vi "SW_Fire_TTL_at_start_universal.vi"(6 "TTL port(s) config to fire":u8, 7 "TTL pulse length, ms":dbl=250.0 format="%#_13g", 8 "error in (no error)":errorcluster, 9 "Serial Port In":refnum<visa-resource-name>="COM3", 10 "Close VISA (T)":bool=TRUE, 11 "Start/stop signaling (F)":bool) -> (0 "error out":errorcluster, 1 "Serial Port Out":refnum<visa-resource-name>="COM3", 3 "Time spent to process command, ms":dbl=250.0)   [LabVIEW 2016]
doc: "Fires TTL High to the TTL2 output for ~250 ms (default)."
uses:
  <vilib>/Instr/_visa.llb/VISA Flush IO Buffer Mask.ctl
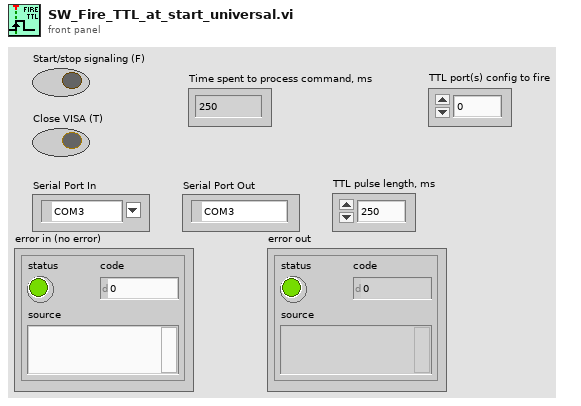
[diagram p1: front panel]
types:
  T1 = typedef "VISA Flush IO Buffer Mask.ctl" = u16
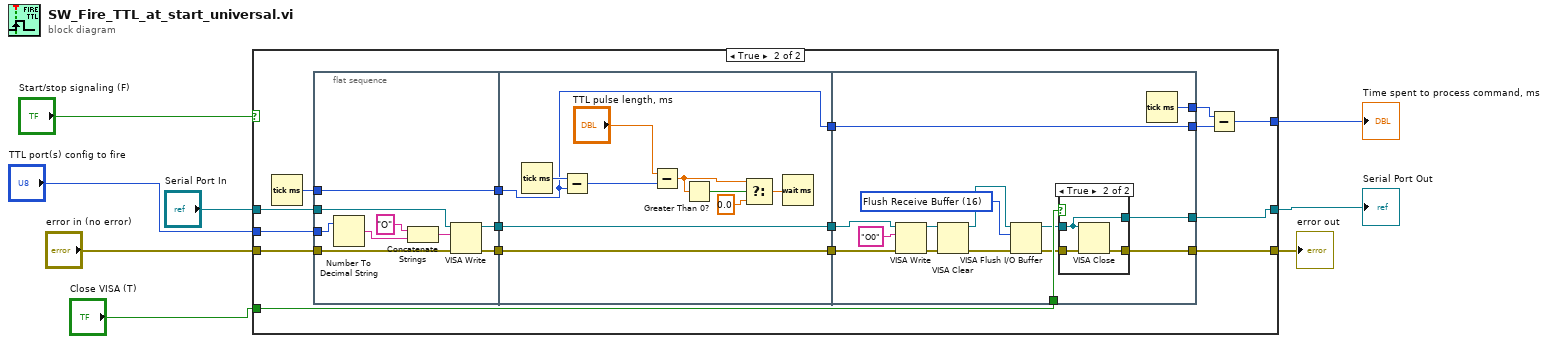
[diagram p0: block diagram]
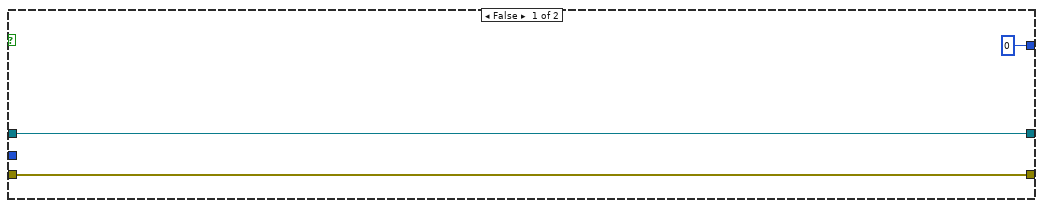
[diagram p2: hidden frame]
diagram:
  n1 = case shown="True" "Start/stop signaling (F)" {
    tunnel: [u32 0 w18] -> w8
    tunnel: [w10 w17] -> w7
    tunnel: "Serial Port In" -> [w10 w16]
    tunnel: "Close VISA (T)" -> [_ w15]
    tunnel: [w9 w14] -> w3
    tunnel: "error in (no error)" -> [w9 w13]
    tunnel: "TTL port(s) config to fire" -> [_ w12]
    frame False {
    }
    frame True {
      n2 = Tick Count (ms)() -> (millisecond timer value=w22:u32)
      n3 = flat-sequence {
        tunnel: w16 -> [w34]
        tunnel: [w36] -> w27
        tunnel: [w35] -> w26
        tunnel: [w33] -> w23
        tunnel: w22 -> [w33]
        tunnel: w13 -> [w32]
        tunnel: w12 -> [w29]
        tunnel: [w46] -> w25
        tunnel: w27 -> [w46]
        tunnel: [w45] -> w24
        tunnel: w26 -> [w45]
        tunnel: w23 -> [w37]
        tunnel: [w37] -> w19
        tunnel: [w58] -> w14
        tunnel: [w59] -> w17
        tunnel: [w60] -> w20
        tunnel: [w61] -> w21
        tunnel: w15 -> [w57]
        tunnel: w19 -> [w60]
        tunnel: w24 -> [w51]
        tunnel: w25 -> [w50]
        frame #0 {
          n4 = Number To Decimal String(number=w29) -> (decimal integer string=w31:string)  [unwired: 1 in]
          n5 = Concatenate Strings("O" ("string"), w31) -> (w28:string)
          n6 = VISA Write(VISA resource name=w34, write buffer=w28, error in (no error)=w32) -> (VISA resource name out=w36:refnum<visa-resource-name>, error out=w35:errorcluster)  [unwired: 1 out]
        }
        frame #1 {
          n7 = Tick Count (ms)() -> (millisecond timer value=w44:u32)
          n8 = Subtract(x=w44, y=w37) -> (x-y=w42:u32)
          n9 = Subtract(x="TTL pulse length, ms", y=w42) -> (x-y=w39:dbl)
          n10 = Greater Than 0?(x=w39) -> (x > 0?=w41:bool)
          n11 = Select(t=w39, s=w41, f=0.0) -> (s? t:f=w40:dbl)
          n12 = Wait (ms)(milliseconds to wait=w40) -> ()  [unwired: 1 out]
        }
        frame #2 {
          w52 = T1 16 items=["Flush Receive Buffer"=16, "Write Transmit Buffer to Device"=32, "Flush Receive Buffer (No I/O)"=64, "Flush Transmit Buffer"=128] ("Mask")
          n13 = VISA Write(VISA resource name=w50, write buffer="O0" ("string"), error in (no error)=w51) -> (VISA resource name out=w49:refnum<visa-resource-name>, error out=w48:errorcluster)  [unwired: 1 out]
          n14 = VISA Clear(VISA resource name=w49, error in (no error)=w48) -> (VISA resource name out=w54:refnum<visa-resource-name>, error out=w56:errorcluster)
          n15 = VISA Flush I/O Buffer(VISA resource name=w54, mask (16)=w52, error in (no error)=w56) -> (VISA resource name out=w53:refnum<visa-resource-name>, error out=w55:errorcluster)
          n16 = case shown="True" w57 {
            tunnel: w53 -> [w63 w65]
            tunnel: w55 -> [w62 w64]
            tunnel: [w63 w65] -> w59
            tunnel: [w62 w66] -> w58
            frame False {
            }
            frame True {
              n17 = VISA Close(VISA resource name=w65, error in (no error)=w64) -> (error out=w66:errorcluster)
            }
          }
          n18 = Tick Count (ms)() -> (millisecond timer value=w61:u32)
        }
      }
      n19 = Subtract(x=w21, y=w20) -> (x-y=w18:u32)
    }
  }
  "Time spent to process command, ms" <- w8
  "Serial Port Out" <- w7
  "error out" <- w3
